vi "SubstituteClusterElementSByLabel.vi"(8 "error in (no error)":errorcluster, 9 "ElementsHyerarchi":string[][](array[string]), 10 "NewElementsValues":variant[](array[variant]), 11 "ClusterIn":variant) -> (0 "error out":errorcluster, 3 "UpdatedCluster out":variant)   [LabVIEW 2013]
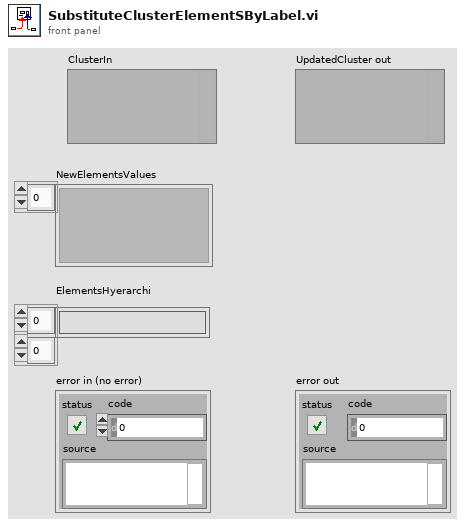
[diagram p1: front panel]
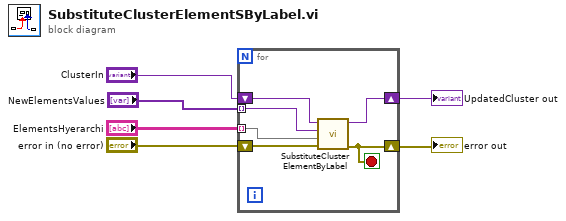
[diagram p0: block diagram]
diagram:
  n1 = for {
    shift-right: [w11] -> w2
    shift-left: "ClusterIn" -> [w10]
    tunnel: "NewElementsValues" -> [w9] mode=indexing
    shift-right: [w8] -> w3
    shift-left: "error in (no error)" -> [w12]
    tunnel: "ElementsHyerarchi" -> [w7] mode=indexing
    stop <- w8 stop-if-true
    n2 = call "SubstituteClusterElementByLabel.vi"("error in (no error)"=w12, "ElementHierarchy"=w7, "NewElementValue"=w9, "ClusterIn"=w10) -> ("ErrorOut"=w8:errorcluster, "UpdatedClusterOut"=w11:variant)  [unwired: 5 in, 1 out]
  }
  "error out" <- w3
  "UpdatedCluster out" <- w2
